vi "3c.vi"() -> ()   [LabVIEW 2014]
panel:
  out "X!":i64
  in  "X":i64
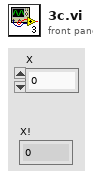
[diagram p1: front panel]
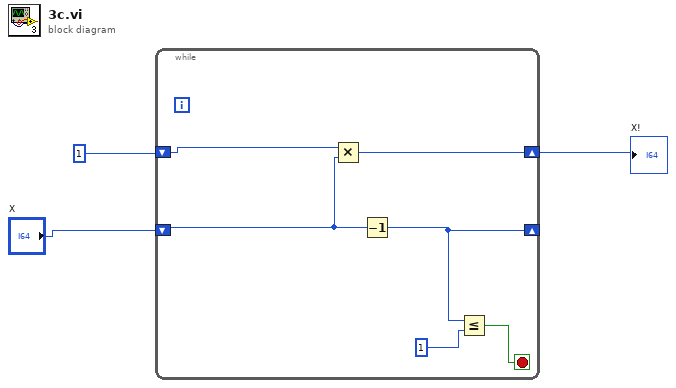
[diagram p0: block diagram]
diagram:
  n1 = while {
    shift-right: [w5] -> w1
    shift-left: 1 -> [w4]
    shift-right: [w7] -> _
    shift-left: "X" -> [w6]
    stop <- w9 stop-if-true
    n2 = Multiply(x=w4, y=w6) -> (x*y=w5:i64)
    n3 = Decrement(x=w6) -> (x-1=w7:i64)
    n4 = Less Or Equal?(x=w7, y=1) -> (x <= y?=w9:bool)
  }
  "X!" <- w1
